vi "Chart[Template].SetParams.vi"(8 "error in (no error)":errorcluster, 10 "ChartParams":T1={"Chart ScaleMultipliers"={"WF Xscale Multiplier"=1000.0, "WF Yscale Multiplier"=[]}, "Coord Transform Multipliers"={"Z-Multiplier"=1.0, "Th-Multiplier"=0.0}}, 11 "DisplayWaveforms":refnum<class "DisplayWaveforms.lvclass">) -> (0 "error out":errorcluster, 3 "DisplayWaveforms out":refnum<class "DisplayWaveforms.lvclass">)   [LabVIEW 2020, in "DisplayWaveform.lvlib" / "DisplayWaveforms.lvclass"]
doc: "---------------------------------------------------------------\nJKI State Machine Objects™\nhttp://jki.net/state-machine-objects/\nCopyright (C) 2005-2015, JKI <info@jki.net>\nALL RIGHTS RESERVEDJKI State Machine Objects (SMO) 1.0.0.5\nJKI - JKI\nCopyright (c) 2016, JKI"
uses:
  DisplayWaveforms.lvclass
  Controller/TypeDefs/ChartParamsCluster.ctl
  DisplayWaveforms.lvclass/DisplayWaveforms.ctl
panel:
  # "For instructions on how to use the JKI State Machine Objects, examples and video tutorials, visit:\nhttp://jki.net/state-machine-objects/\n\nJKI State Machine Objects™\nhttp://jki.net/state-machine-objects/\nCopyright (C) 2005-2015, JKI <info@jki.net>\nALL RIGHTS RESERVED"
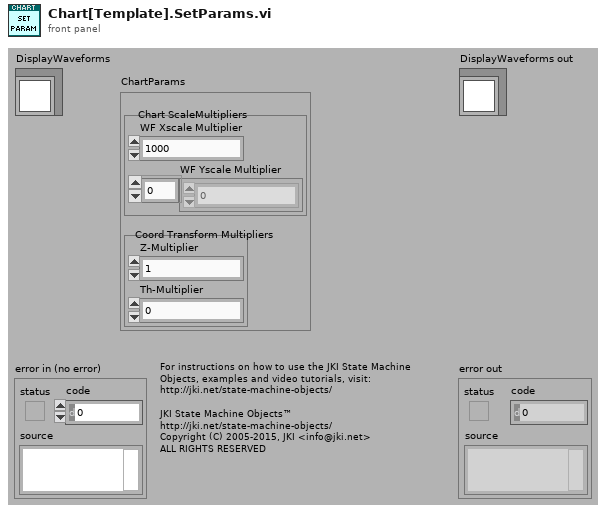
[diagram p1: front panel]
types:
  T1 = typedef "ChartParamsCluster.ctl" = cluster{"Chart ScaleMultipliers":cluster{"WF Xscale Multiplier":dbl, "WF Yscale Multiplier":dbl[]}, "Coord Transform Multipliers":cluster{"Z-Multiplier":dbl, "Th-Multiplier":dbl}}
  T2 = typedef "DisplayWaveform.lvlib/DisplayWaveforms.lvclass/PublicEvents--Cluster.ctl" = cluster{"Chart Cleared":refnum<user-event>, "Chart Exported":refnum<user-event>, "ChartParams Set":refnum<user-event>}
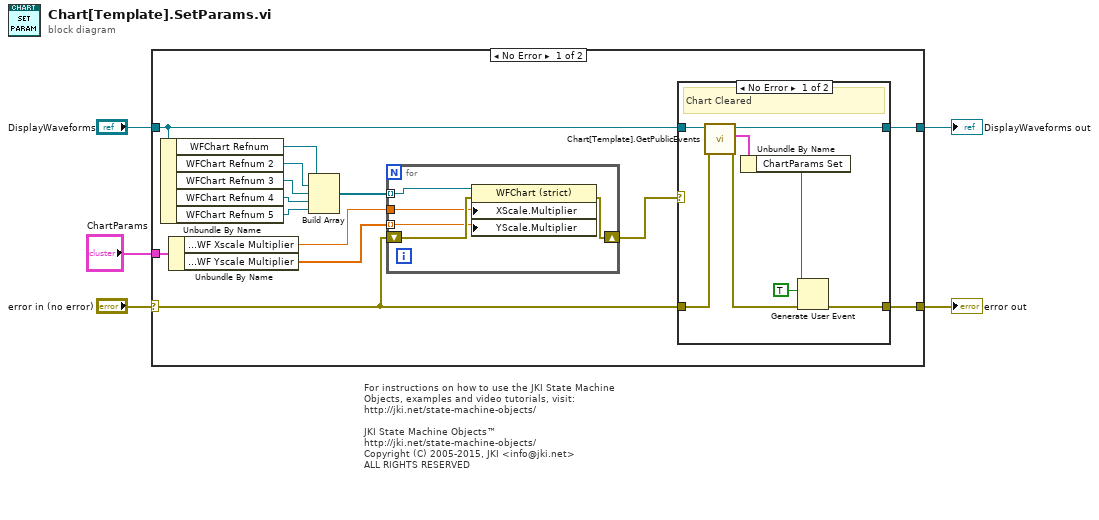
[diagram p0: block diagram]
diagram:
  # "For instructions on how to use the JKI State Machine Objects, examples and video tutorials, visit:\nhttp://jki.net/state-machine-objects/\n\nJKI State Machine Objects™\nhttp://jki.net/state-machine-objects/\nCopyright (C) 2005-2015, JKI <info@jki.net>\nALL RIGHTS RESERVED"
  n1 = case shown="No Error" "error in (no error)" {
    selector: "error in (no error)" -> [w9 w35]
    tunnel: "DisplayWaveforms" -> [w16 w36]
    tunnel: [w19 w35] -> w4
    tunnel: [w18 w36] -> w3
    tunnel: "ChartParams" -> [w8 _]
    frame No Error {
      n2 = Unbundle By Name(w16) -> ("WFChart Refnum"=w15:refnum<vi>, "WFChart Refnum 2"=w14:refnum<vi>, "WFChart Refnum 3"=w13:refnum<vi>, "WFChart Refnum 4"=w12:refnum<vi>, "WFChart Refnum 5"=w11:refnum<vi>)
      n3 = Unbundle By Name(w8) -> ("Chart ScaleMultipliers.WF Xscale Multiplier"=w7:dbl, "Chart ScaleMultipliers.WF Yscale Multiplier"=w6:dbl[])
      n4 = Build Array(w15, w14, w13, w12, w11) -> (w10:refnum<vi>[])
      n5 = for {
        tunnel: w10 -> [w23] mode=indexing
        shift-right: [w24] -> w17
        shift-left: w9 -> [w22]
        tunnel: w7 -> [w21]
        tunnel: w6 -> [w20] mode=indexing
        n6 = property class="WFChart (strict)"(reference=w23, error in=w22, "XScale.Multiplier"=w21, "YScale.Multiplier"=w20) -> (error out=w24:errorcluster)  [unwired: 1 out]
      }
      n7 = case shown="No Error" w17 {
        tunnel: w9 -> [w30 w33]
        tunnel: [w27 w33] -> w19
        tunnel: w16 -> [w32 w34]
        tunnel: [w31 w34] -> w18
        frame No Error {
          # "Chart Cleared"
          n8 = call "Chart[Template].GetPublicEvents.vi"("error in (no error)"=w30, "DisplayWaveforms"=w32) -> ("error out"=w28:errorcluster, "Chart[Template] Public Events"=w29:T2, "DisplayWaveforms out"=w31:refnum<class "DisplayWaveforms.lvclass">)  [unwired: 7 in]
          n9 = Unbundle By Name(w29) -> ("ChartParams Set"=w25:refnum<user-event>)
          n10 = Generate User Event(user event=w25, event data cluster=TRUE ("event data"), error in=w28) -> (error out=w27:errorcluster)  [unwired: 1 in, 1 out]
        }
        frame Error {
          # "Chart was not cleared"
        }
      }
    }
    frame Error {
    }
  }
  "error out" <- w4
  "DisplayWaveforms out" <- w3
